vi "Wakeup Message.vi"(8 "error in (no error)":errorcluster, 10 "Wakeup Bit (Set)":cluster{"Address":u16, "Set/Reset":bool}, 11 "Signal Acquisition in":refnum<class "Signal Acquisition.lvclass">) -> (0 "error out":errorcluster, 3 "Signal Acquisition out":refnum<class "Signal Acquisition.lvclass">)   [LabVIEW 2022 SP3]
uses:
  Signal Acquisition.lvclass
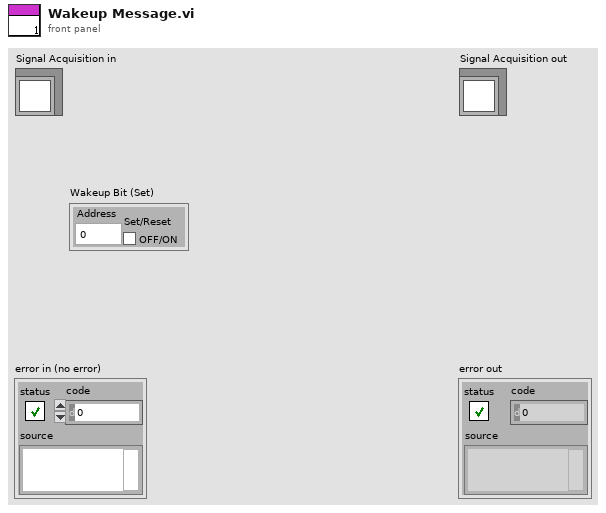
[diagram p1: front panel]
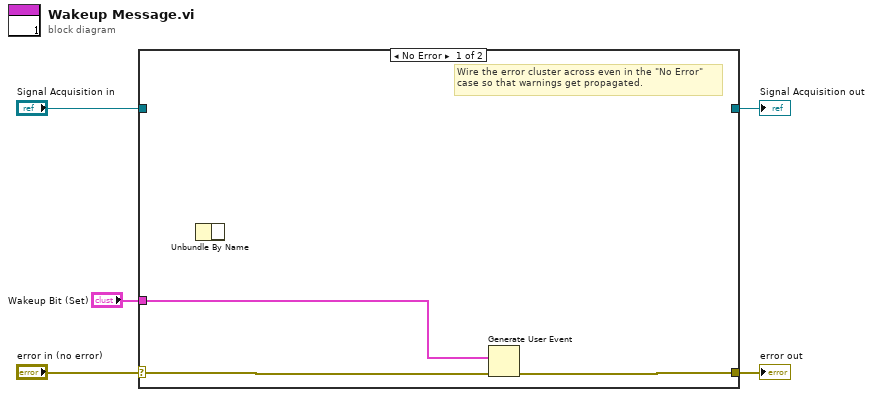
[diagram p0: block diagram]
diagram:
  n1 = case shown="No Error" "error in (no error)" {
    selector: "error in (no error)" -> [w8 w10]
    tunnel: [w7 w10] -> w4
    tunnel: [_ w9] -> w2
    tunnel: "Signal Acquisition in" -> [_ w9]
    tunnel: "Wakeup Bit (Set)" -> [w6 _]
    frame No Error {
      # "Wire the error cluster across even in the \"No Error\"\ncase so that warnings get propagated."
      n2 = Unbundle By Name() -> ()  [unwired: 1 in, 1 out]
      n3 = Generate User Event(event data cluster=w6, error in=w8) -> (error out=w7:errorcluster)  [unwired: 2 in, 1 out]
    }
    frame Error {
    }
  }
  "error out" <- w4
  "Signal Acquisition out" <- w2
